vi "Read ColorSelectorBackground.vi"(8 "error in (no error)":errorcluster, 11 "Calendar in":refnum<class "Calendar.lvclass">) -> (0 "error out":errorcluster, 2 "ColorSelectorBackground":u32(colorbox), 3 "Calendar out":refnum<class "Calendar.lvclass">)   [LabVIEW 2015, in "Calendar.lvclass"]
uses:
  Calendar.lvclass
  Calendar.lvclass/Calendar.ctl
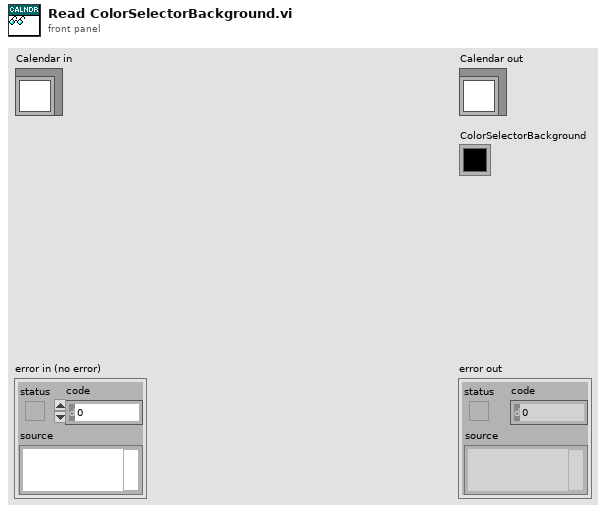
[diagram p1: front panel]
types:
  T1 = typedef "Calendar.lvclass/State Data.ctl" = cluster{"Current Date":timestamp, "First Day of Week":T2, "Color":cluster{"Selector Background":u32, "Selector Text":u32, "Days of Week Background":u32, "Days of Week Text":u32, "Calendar Background":u32, "Calendar Text":u32, "Calendar Selection Background":u32, "Calendar Selection Text":u32}, "Visible":cluster{"Today Selector Visible":bool, "Month-Year Selector Visible":bool}}
  T2 = typedef "Calendar.lvclass/DaysOfWeek.ctl" = enum16{"Sunday", "Monday", "Tuesday", "Wednesday", "Thursday", "Friday", "Saturday"}
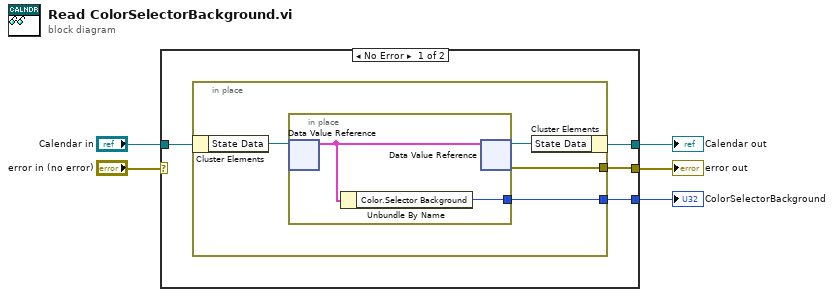
[diagram p0: block diagram]
diagram:
  n1 = case shown="No Error" "error in (no error)" {
    selector: "error in (no error)" -> [_ w17]
    tunnel: [w7 w17] -> w4
    tunnel: [w8 w16] -> w2
    tunnel: "Calendar in" -> [w9 w16]
    tunnel: [w6 _] -> w1
    frame No Error {
      n2 = in-place {
        in-place-border: [w11] -> w7
        in-place-border: [w10] -> w6
        n3 = in-place-cluster #1(w9) -> ("State Data"=w13:refnum<data-value>)
        n4 = in-place {
          in-place-border: [w14] -> w10
          n5 = in-place-dvr #2(w13) -> (w15:T1)  [unwired: 1 out]
          n6 = Unbundle By Name(w15) -> ("Color.Selector Background"=w14:u32)
          n7 = in-place-dvr #2(w15) -> (w12:refnum<data-value>, w11:errorcluster)
        }
        n8 = in-place-cluster #1("State Data"=w12) -> (w8:refnum<class "Calendar.lvclass">)
      }
    }
    frame Error {
    }
  }
  "error out" <- w4
  "Calendar out" <- w2
  "ColorSelectorBackground" <- w1
